vi "Calculate Corner Coordinates (SubVI).vi"() -> (20 "lcx1":dbl, 21 "lcy1":dbl, 22 "rcx1":dbl, 23 "rcy1":dbl, 24 "lcx2":dbl, 25 "lcy2":dbl, 26 "rcx2":dbl, 27 "rcy2":dbl)   [LabVIEW 2015]
uses:
  Left Variables.vi
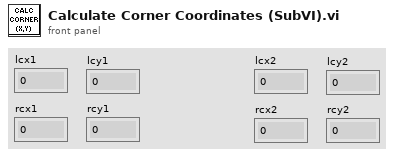
[diagram p1: front panel]
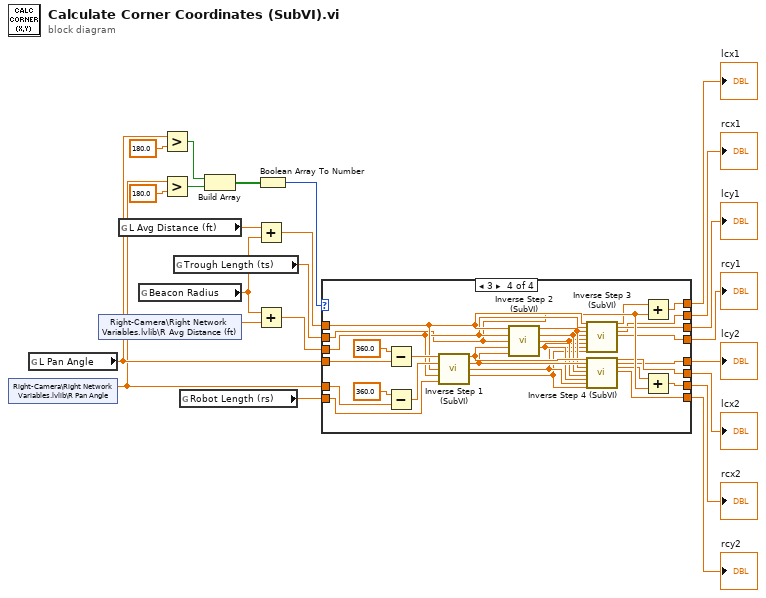
[diagram p0: block diagram]
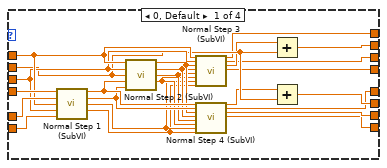
[diagram p2: hidden frame]
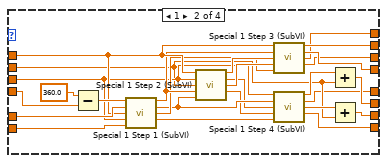
[diagram p3: hidden frame]
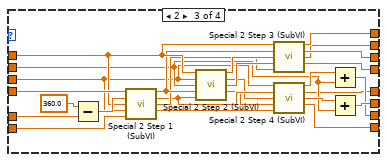
[diagram p4: hidden frame]
diagram:
  n1 = shared-variable "Right-Camera\\Right Network Variables.lvlib\\R Pan Angle"() -> (w13:dbl)  [unwired: 1 in, 1 out]
  n2 = global read "Left Variables.vi" "L Pan Angle"() -> (w14:dbl)
  n3 = shared-variable "Right-Camera\\Right Network Variables.lvlib\\R Avg Distance (ft)"() -> (w18:dbl)  [unwired: 1 in, 1 out]
  n4 = global read "Left Variables.vi" "L Avg Distance (ft)"() -> (w22:dbl)
  n5 = global read "Left Variables.vi" "Beacon Radius"() -> (w19:dbl)
  n6 = Greater?(x=w14, y=180.0) -> (0:w12:bool)
  n7 = Greater?(x=w13, y=180.0) -> (0:w11:bool)
  n8 = global read "Left Variables.vi" "Trough Length (ts)"() -> (w17:dbl)
  n9 = global read "Left Variables.vi" "Robot Length (rs)"() -> (w23:dbl)
  n10 = Build Array(w12, w11) -> (w10:bool[])
  n11 = Add(x=w22, y=w19) -> (x+y=w21:dbl)
  n12 = Add(x=w19, y=w18) -> (x+y=w20:dbl)
  n13 = Boolean Array To Number(Boolean array=w10) -> (number=w9:u32)
  n14 = case shown="3" w9 {
    tunnel: w14 -> [w46 w72 w95 w125]
    tunnel: w13 -> [w45 w70 w98 w124]
    tunnel: w23 -> [w47 w69 w97 w121]
    tunnel: w21 -> [w44 w68 w94 w120]
    tunnel: w20 -> [w43 w59 w78 w119]
    tunnel: w17 -> [w34 w52 w83 w110]
    tunnel: [w31 w51 w82 w102] -> w8
    tunnel: [w30 w49 w80 w101] -> w7
    tunnel: [w29 w50 w81 w108] -> w6
    tunnel: [w28 w48 w79 w100] -> w5
    tunnel: [w27 w61 w89 w109] -> w4
    tunnel: [w26 w60 w88 w105] -> w3
    tunnel: [w25 w63 w87 w104] -> w2
    tunnel: [w24 w62 w86 w103] -> w1
    frame 0, Default {
      n15 = call "Normal Step 1 (SubVI).vi"("aLC"=w46, "aRC"=w45, "Ldist"=w44, "Rdist"=w43, "Rside"=w47) -> ("lbrc"=w42:dbl, "rblc"=w41:dbl, "aLB2"=w36:dbl, "aRB2"=w35:dbl)  [unwired: 7 in]
      n16 = call "Normal Step 2 (SubVI).vi"("Ldist"=w44, "Rdist"=w43, "Tside"=w34, "lbrc"=w42, "rblc"=w41) -> ("aLB"=w40:dbl, "aRB"=w39:dbl, "aLB1"=w38:dbl, "aRB1"=w37:dbl)  [unwired: 7 in]
      n17 = call "Normal Step 3 (SubVI).vi"("Ldist"=w44, "Rdist"=w43, "aLB"=w40, "aRB"=w39, "aLB1"=w38, "aRB1"=w37, "aLB2"=w36, "aRB2"=w35) -> ("lcx1"=w27:dbl, "lcy1"=w26:dbl, "rcx1"=w33:dbl, "rcy1"=w24:dbl)  [unwired: 14 in, 2 out]
      n18 = call "Normal Step 4 (SubVI).vi"("lbrc"=w42, "rblc"=w41, "aLB"=w40, "aRB"=w39, "aLB1"=w38, "aRB1"=w37, "aLB2"=w36, "aRB2"=w35) -> ("lcx2"=w32:dbl, "lcy2"=w30:dbl, "rcx2"=w29:dbl, "rcy2"=w28:dbl)  [unwired: 14 in, 2 out]
      n19 = Add(x=w33, y=w34) -> (x+y=w25:dbl)
      n20 = Add(x=w32, y=w34) -> (x+y=w31:dbl)
    }
    frame 1 {
      n21 = Subtract(x=360.0, y=w72) -> (x-y=w71:dbl)
      n22 = call "Special 1 Step 1 (SubVI).vi"("aLC"=w71, "aRC"=w70, "Ldist"=w68, "Rdist"=w59, "Rside"=w69) -> ("lbrc"=w67:dbl, "rblc"=w58:dbl, "aLB2"=w64:dbl, "aRB2"=w55:dbl)  [unwired: 7 in]
      n23 = call "Special 1 Step 2 (SubVI).vi"("Ldist"=w68, "Rdist"=w59, "Tside"=w52, "lbrc"=w67, "rblc"=w58) -> ("aLB"=w66:dbl, "aRB"=w57:dbl, "aLB1"=w65:dbl, "aRB1"=w56:dbl)  [unwired: 7 in]
      n24 = call "Special 1 Step 3 (SubVI).vi"("Ldist"=w68, "lbrc"=w67, "aLB"=w66, "aLB1"=w65, "aLB2"=w64) -> ("rcx1"=w63:dbl, "rcy1"=w62:dbl, "lcx1"=w61:dbl, "lcy1"=w60:dbl)  [unwired: 6 in, 1 out]
      n25 = call "Special 1 Step 4 (SubVI).vi"("Rdist"=w59, "rblc"=w58, "aRB"=w57, "aRB1"=w56, "aRB2"=w55) -> ("lcx2"=w54:dbl, "lcy2"=w49:dbl, "rcx2"=w53:dbl, "rcy2"=w48:dbl)  [unwired: 6 in, 1 out]
      n26 = Add(x=w54, y=w52) -> (x+y=w51:dbl)
      n27 = Add(x=w53, y=w52) -> (x+y=w50:dbl)
    }
    frame 2 {
      n28 = Subtract(x=360.0, y=w98) -> (x-y=w96:dbl)
      n29 = call "Special 2 Step 1 (SubVI).vi"("aLC"=w95, "aRC"=w96, "Ldist"=w94, "Rdist"=w78, "Rside"=w97) -> ("lbrc"=w93:dbl, "rblc"=w77:dbl, "aLB2"=w90:dbl, "aRB2"=w74:dbl)  [unwired: 7 in]
      n30 = call "Special 2 Step 2 (SubVI).vi"("Ldist"=w94, "Rdist"=w78, "Tside"=w83, "lbrc"=w93, "rblc"=w77) -> ("aLB"=w92:dbl, "aRB"=w76:dbl, "aLB1"=w91:dbl, "aRB1"=w75:dbl)  [unwired: 7 in]
      n31 = call "Special 2 Step 3 (SubVI).vi"("Ldist"=w94, "lbrc"=w93, "aLB"=w92, "aLB1"=w91, "aLB2"=w90) -> ("lcx1"=w89:dbl, "lcy1"=w88:dbl, "rcx1"=w87:dbl, "rcy1"=w86:dbl)  [unwired: 6 in, 1 out]
      n32 = call "Special 2 Step 4 (SubVI).vi"("Rdist"=w78, "rblc"=w77, "aRB"=w76, "aRB1"=w75, "aRB2"=w74) -> ("lcx2"=w85:dbl, "lcy2"=w80:dbl, "rcx2"=w84:dbl, "rcy2"=w79:dbl)  [unwired: 6 in, 1 out]
      n33 = Add(x=w85, y=w83) -> (x+y=w81:dbl)
      n34 = Add(x=w84, y=w83) -> (x+y=w82:dbl)
    }
    frame 3 {
      n35 = Subtract(x=360.0, y=w125) -> (x-y=w123:dbl)
      n36 = Subtract(x=360.0, y=w124) -> (x-y=w122:dbl)
      n37 = call "Inverse Step 1 (SubVI).vi"("aLC"=w123, "aRC"=w122, "Ldist"=w120, "Rdist"=w119, "Rside"=w121) -> ("lblc"=w118:dbl, "rbrc"=w117:dbl, "aLB2"=w112:dbl, "aRB2"=w111:dbl)  [unwired: 7 in]
      n38 = call "Inverse Step 2 (SubVI).vi"("Ldist"=w120, "Rdist"=w119, "Tside"=w110, "lblc"=w118, "rbrc"=w117) -> ("aLB"=w116:dbl, "aRB"=w115:dbl, "aLB1"=w114:dbl, "aRB1"=w113:dbl)  [unwired: 7 in]
      n39 = call "Inverse Step 3 (SubVI).vi"("Ldist"=w120, "Rdist"=w119, "aLB"=w116, "aRB"=w115, "aLB1"=w114, "aRB1"=w113, "aLB2"=w112, "aRB2"=w111) -> ("lcx1"=w106:dbl, "lcy1"=w105:dbl, "rcx1"=w104:dbl, "rcy1"=w103:dbl)  [unwired: 14 in, 2 out]
      n40 = call "Inverse Step 4 (SubVI).vi"("lblc"=w118, "rbrc"=w117, "aLB"=w116, "aRB"=w115, "aLB1"=w114, "aRB1"=w113, "aLB2"=w112, "aRB2"=w111) -> ("lcx2"=w102:dbl, "lcy2"=w101:dbl, "rcx2"=w107:dbl, "rcy2"=w100:dbl)  [unwired: 14 in, 2 out]
      n41 = Add(x=w106, y=w110) -> (x+y=w109:dbl)
      n42 = Add(x=w107, y=w110) -> (x+y=w108:dbl)
    }
  }
  "lcx2" <- w8
  "lcy2" <- w7
  "rcx2" <- w6
  "rcy2" <- w5
  "lcx1" <- w4
  "lcy1" <- w3
  "rcx1" <- w2
  "rcy1" <- w1
